vi "Get Transfer Notifier.vi"(8 "error in":errorcluster, 11 "SDO Transfer in":refnum<class "SDO Transfer.lvclass">) -> (0 "error out":errorcluster, 2 "SDO Transfer Notifier":refnum<notifier>, 3 "SDO Transfer out":refnum<class "SDO Transfer.lvclass">)   [LabVIEW 2020, in "CANopen.lvlib" / "SDO Manager.lvlib" / "SDO Transfer.lvclass"]
uses:
  SDO Transfer.lvclass
  SDO Transfer.lvclass/SDO Transfer.ctl
  SDO abort code.ctl
  Typedefs/SDO Result.ctl
  SDO Transfer Result.ctl
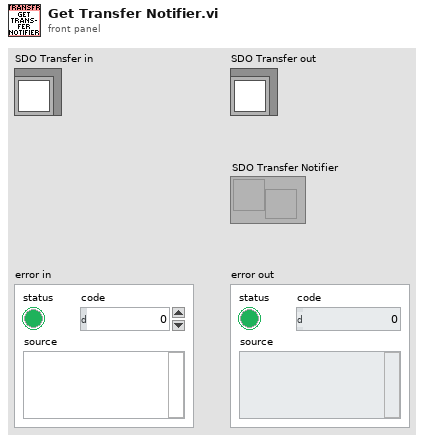
[diagram p1: front panel]
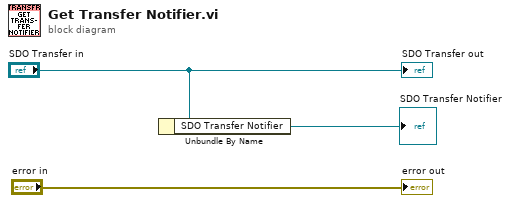
[diagram p0: block diagram]
diagram:
  n1 = Unbundle By Name("SDO Transfer in") -> ("SDO Transfer Notifier"=→"SDO Transfer Notifier":refnum<notifier>)
  "error out" <- "error in"
  "SDO Transfer out" <- "SDO Transfer in"
